vi "multiply_array.vi"() -> ()   [LabVIEW 2020]
panel:
  out "error out":errorcluster
  in  "Library Path":path=path "/home/saman/src/lvcc/build/test/libtest.so"
  in  "no":i32=2
  in  "arr 2":i32[](array[numeric])=[1, 2, 3]
  out "arr":i32[](array[numeric])=[2, 4, 6]
  # "x"
  # "="
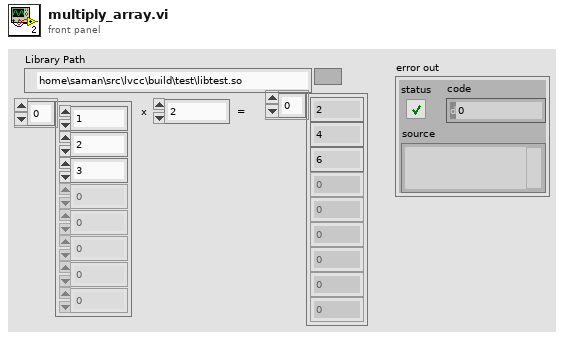
[diagram p1: front panel]
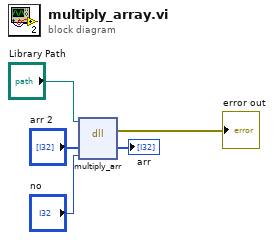
[diagram p0: block diagram]
diagram:
  n1 = dll-call lib="home/saman/src/lvcc/build/test/libtest.so" fn="multiply_arr"(path in="Library Path", "arr"="arr 2", "no"="no") -> (error out=→"error out":errorcluster, "arr"=→"arr":i32[])  [unwired: 4 in, 1 out]
